vi "ATM.vi"() -> ()   [LabVIEW 2018]
panel:
  in  "stop":bool
  in  "?":bool
  out "balance":dbl
  in  "?":bool
  in  "amount":dbl
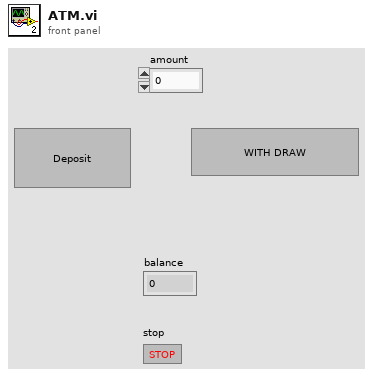
[diagram p1: front panel]
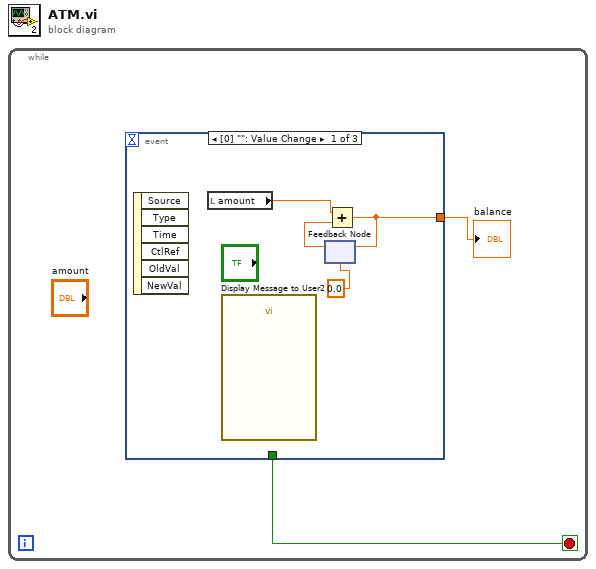
[diagram p0: block diagram]
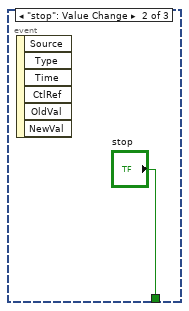
[diagram p2: hidden frame]
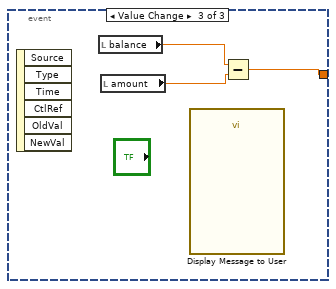
[diagram p3: hidden frame]
diagram:
  n1 = while {
    stop <- w1 stop-if-true
    n2 = event shown="[0] \"\": Value Change" {
      selector: _ -> [_ _ _]
      dyn-events: _ -> [_ _ _]
      timeout: _ -> [_ _ _]
      tunnel: [w4 _ w8] -> w2
      tunnel: [_ "stop" _] -> w1
      event Value Change {
        n3 = event-data() -> ()  [unwired: 1 in, 6 out]
        n4 = local read "amount"() -> (w6:dbl)
        n5 = call "Display Message to User2"() -> ()  [unwired: 10 in, 2 out]
        n6 = feedback #1(0.0) -> (w5:dbl)
        n7 = Add(x=w6, y=w5) -> (x+y=w4:dbl)
        n8 = feedback-in #1(w4) -> ()
      }
      event "stop": Value Change {
        n9 = event-data() -> ()  [unwired: 1 in, 6 out]
      }
      event Value Change {
        n10 = event-data() -> ()  [unwired: 1 in, 6 out]
        n11 = local read "balance"() -> (w10:dbl)
        n12 = local read "amount"() -> (w9:dbl)
        n13 = call "Display Message to User"() -> ()  [unwired: 10 in, 2 out]
        n14 = Subtract(x=w10, y=w9) -> (x-y=w8:dbl)
      }
    }
    "balance" <- w2
  }
